vi "Write Timeout (60000 ms).vi"(8 "error in (no error)":errorcluster, 10 "Timeout (60000 ms)":i32=60000, 11 "WebSocket Client in":refnum<class "WebSocket Client.lvclass">) -> (0 "error out":errorcluster, 3 "WebSocket Client out":refnum<class "WebSocket Client.lvclass">)   [LabVIEW 2016, in "WebSocket Actors.lvlib" / "WebSocket Client.lvclass"]
uses:
  WebSocket Client.lvclass
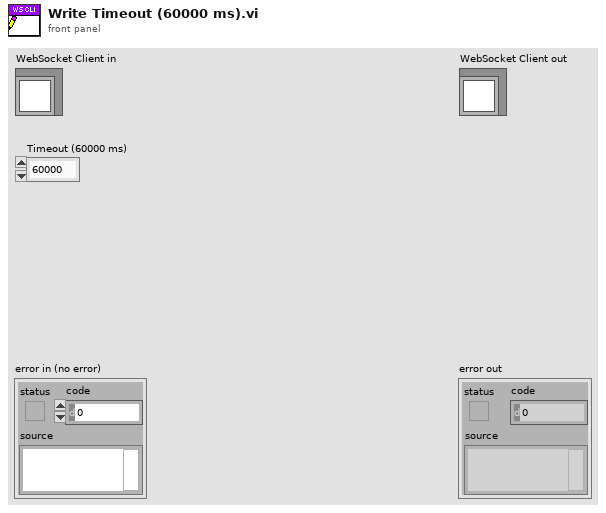
[diagram p1: front panel]
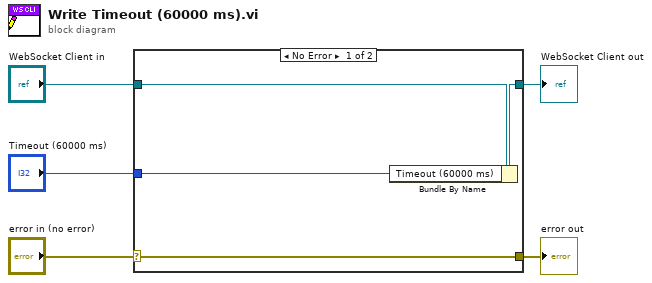
[diagram p0: block diagram]
diagram:
  n1 = case shown="No Error" "error in (no error)" {
    selector: "error in (no error)" -> [w9 w10]
    tunnel: [w9 w10] -> w4
    tunnel: [w7 w11] -> w2
    tunnel: "WebSocket Client in" -> [w8 w11]
    tunnel: "Timeout (60000 ms)" -> [w6 _]
    frame No Error {
      n2 = Bundle By Name(cluster=w8, "Timeout (60000 ms)"=w6) -> (w7:refnum<class "WebSocket Client.lvclass">)
    }
    frame Error {
    }
  }
  "error out" <- w4
  "WebSocket Client out" <- w2
